vi "Get Next Data.vi"(8 "error in (no error)":errorcluster, 11 "Counter Data Plugin in":refnum<class "Counter Data Plugin.lvclass">) -> (0 "error out":errorcluster, 2 "Data":dbl, 3 "Counter Data Plugin out":refnum<class "Counter Data Plugin.lvclass">)   [LabVIEW 2017, in "Data Engine.lvlib" / "Counter Data Plugin.lvclass"]
uses:
  Counter Data Plugin.lvclass
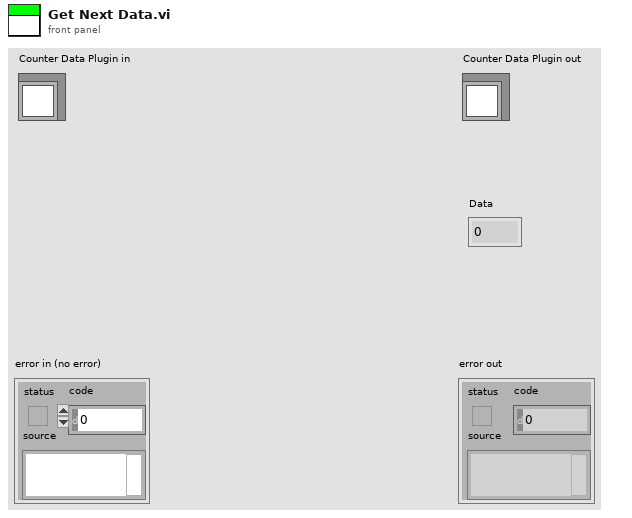
[diagram p1: front panel]
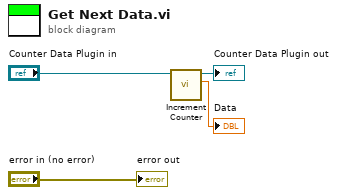
[diagram p0: block diagram]
diagram:
  n1 = call "Increment Counter.vi"("Counter Data Plugin in"="Counter Data Plugin in") -> ("Counter"=→"Data":dbl, "Counter Data Plugin out"=→"Counter Data Plugin out":refnum<class "Counter Data Plugin.lvclass">)  [unwired: 9 in]
  "error out" <- "error in (no error)"
